vi "shift.vi"(10 "Enum":enum16{"forward", "reverse"}(ring)) -> ()   [LabVIEW 2014]
uses:
  <vilib>/Rock Robotics/WPI/Solenoid/WPI_SolenoidValue.ctl
  <vilib>/Rock Robotics/WPI/Solenoid/WPI_SolenoidSetEnum.vi
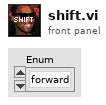
[diagram p1: front panel]
types:
  T1 = typedef "WPI_SolenoidValue.ctl" = enum16{"Off", "On", "Forward", "Reverse"}
  T2 = typedef "WPI_SolenoidDevRef.ctl" = cluster{"DevStatus":errorcluster, "Pneumatics Control Module":u8, "Forward Solenoid Channel":T3, "Reverse Solenoid Channel":T3}
  T3 = typedef "WPI_SolenoidChannel.ctl" = enum8{"Solenoid 0", "Solenoid 1", "Solenoid 2", "Solenoid 3", "Solenoid 4", "Solenoid 5", "Solenoid 6", "Solenoid 7", "Invalid"}
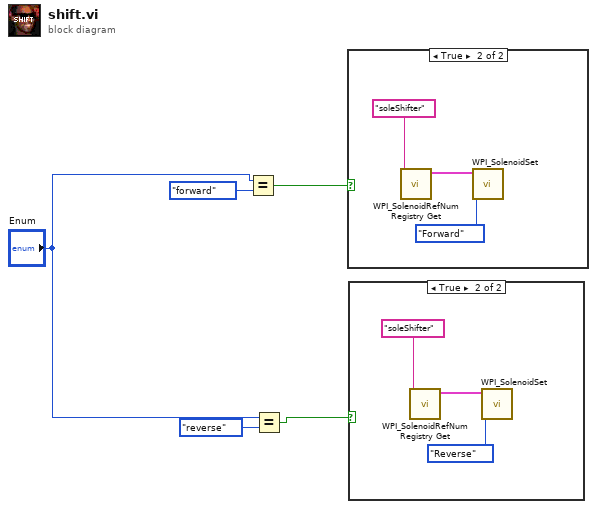
[diagram p0: block diagram]
diagram:
  n1 = Equal?(x="Enum", y=enum16{"forward", "reverse"}."forward") -> (x = y?=w1:bool)
  n2 = Equal?(x="Enum", y=enum16{"forward", "reverse"}."reverse") -> (x = y?=w2:bool)
  n3 = case shown="True" w1 {
    frame False {
    }
    frame True {
      n4 = call <vilib>:"WPI_SolenoidRefNum Registry Get.vi"("refnum name"="soleShifter") -> ("SolenoidDevRef"=w7:T2)  [unwired: 9 in, 1 out]
      n5 = call-poly <vilib>:"WPI_SolenoidSet.vi"("Value"=WPI_SolenoidValue."Forward", "SolenoidDevRef"=w7) -> ()  [unwired: 8 in, 2 out]
    }
  }
  n6 = case shown="True" w2 {
    frame False {
    }
    frame True {
      n7 = call <vilib>:"WPI_SolenoidRefNum Registry Get.vi"("refnum name"="soleShifter") -> ("SolenoidDevRef"=w10:T2)  [unwired: 9 in, 1 out]
      n8 = call-poly <vilib>:"WPI_SolenoidSet.vi"("Value"=WPI_SolenoidValue."Reverse", "SolenoidDevRef"=w10) -> ()  [unwired: 8 in, 2 out]
    }
  }
